vi "Create Result.vi"(8 "error in (no error)":errorcluster, 11 "GObject":refnum<vi>) -> (0 "error out":errorcluster, 3 "Search Result out":refnum<class "Search Result.lvclass">)   [LabVIEW 2016, in "Better Search.lvlib" / "Search Result.lvclass"]
uses:
  Search Result.lvclass
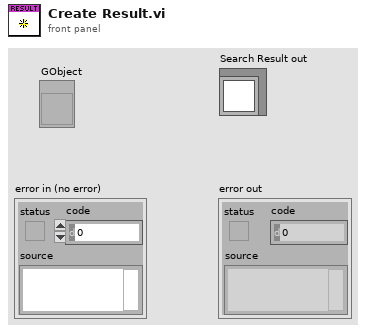
[diagram p1: front panel]
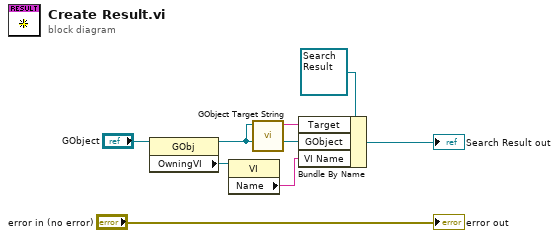
[diagram p0: block diagram]
diagram:
  n1 = property class="GObj"(reference="GObject") -> (reference out=w1:refnum<vi>, "OwningVI"=w4:refnum<vi>)  [unwired: 1 in, 1 out]
  n2 = property class="VI"(reference=w4) -> ("Name"=w3:string)  [unwired: 1 in, 2 out]
  n3 = call "GObject Target String.vi"("GObject"=w1) -> ("Target"=w2:string)  [unwired: 10 in]
  n4 = Bundle By Name(cluster=refnum<class "Search Result.lvclass"> refnum ("Search Result in"), "Target"=w2, "GObject"=w1, "VI Name"=w3) -> (→"Search Result out":refnum<class "Search Result.lvclass">)
  "error out" <- "error in (no error)"
